vi "get waveplate status.vi"(8 "error in (no error)":errorcluster, 11 "Channel in":refnum<class "ECHARPE_Channel.lvclass">) -> (0 "error out":errorcluster, 2 "wp condition":string, 3 "Channel out":refnum<class "ECHARPE_Channel.lvclass">)   [LabVIEW 2018, in "ECHARPE_Channel.lvclass"]
uses:
  ECHARPE_Channel.lvclass
  Server/Server.lvclass/Server.ctl
  RxTx/RxTx.lvclass
  Server/Server.lvclass
panel:
  in  "Cluster":T1
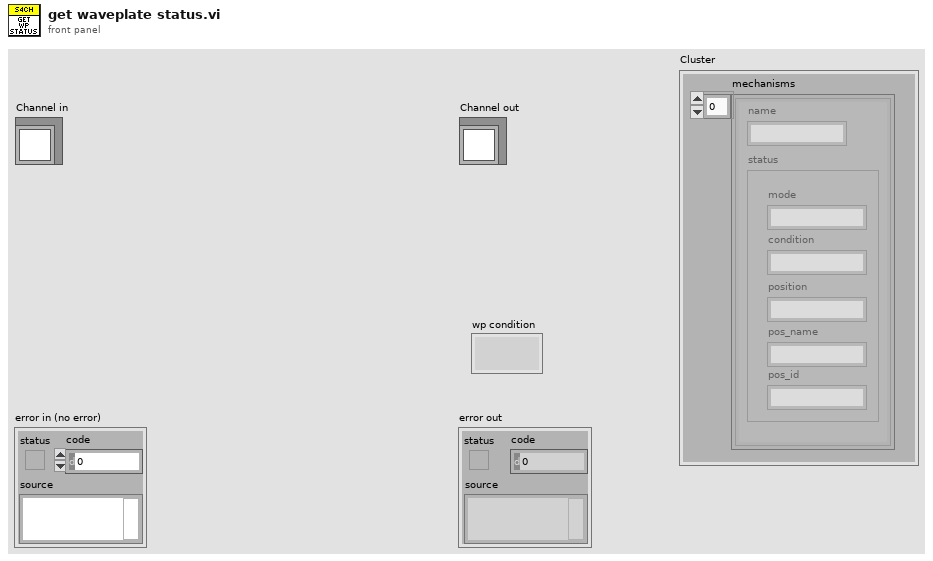
[diagram p1: front panel]
types:
  T1 = cluster{"mechanisms":cluster{"name":string, "status":cluster{"mode":string, "condition":string, "pos_name":string, "position":string, "pos_id":string}}[]}
  T2 = cluster{"State Machine.lvclass":refnum<class "State Machine.lvclass">, "RxTx.lvclass":refnum<class "RxTx.lvclass">, "Save_Header_RxTx.lvclass":refnum<class "RxTx.lvclass">, "Status SM.lvclass":refnum<class "State Machine.lvclass">, "Status RxTx.lvclass":refnum<class "RxTx.lvclass">, "servers array":refnum<class "Server.lvclass">[], "Events log file.lvclass":refnum<class "Log File.lvclass">, "Errors log file.lvclass":refnum<class "Log File.lvclass">, "Keywords log file.lvclass":refnum<class "Log File.lvclass">, "Sim_CCD.lvclass":refnum<class "Sim_CCD.lvclass">}
  T3 = cluster{"name":string, "status":cluster{"mode":string, "condition":string, "pos_name":string, "position":string, "pos_id":string}}[]
  T4 = cluster{"name":string, "status":cluster{"mode":string, "condition":string, "pos_name":string, "position":string, "pos_id":string}}
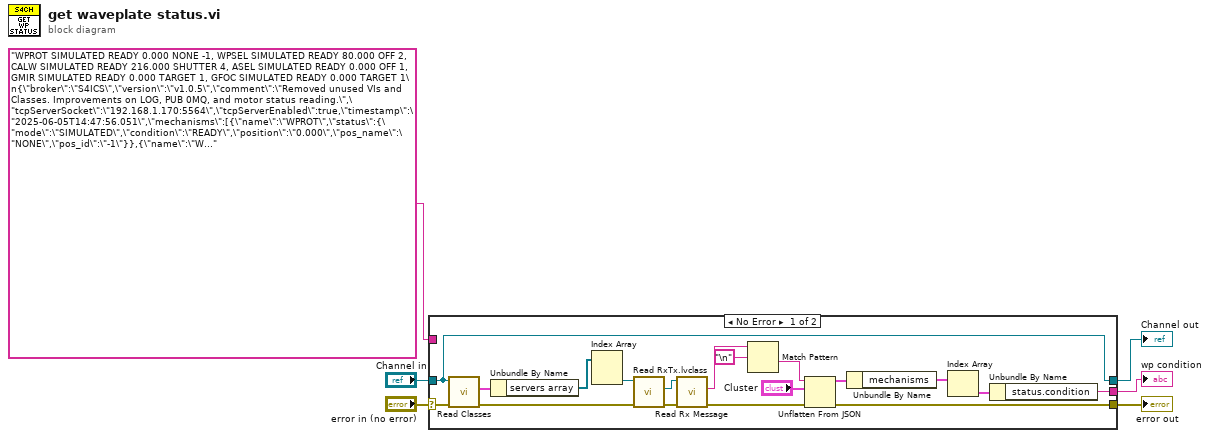
[diagram p0: block diagram]
diagram:
  n1 = case shown="No Error" "error in (no error)" {
    selector: "error in (no error)" -> [w11 w26]
    tunnel: [w24 w26] -> w5
    tunnel: [w10 w25] -> w3
    tunnel: "Channel in" -> [w10 w25]
    tunnel: [w14 _] -> w2
    tunnel: "WPROT SIMULATED READY 0.000 NONE -1, WPSEL SIMULATED READY 80.000 OFF 2, CALW SIMULATED READY 216.000 SHUTTER 4, ASEL SIMULATED READY 0.000 OFF 1, GMIR SIMULATED READY 0.000 TARGET 1, GFOC SIMULATED READY 0.000 TARGET 1\n{\"broker\":\"S4ICS\",\"version\":\"v1.0.5\",\"comment\":\"Removed unused VIs and Classes. Improvements on LOG, PUB 0MQ, and motor status reading.\",\"tcpServerSocket\":\"192.168.1.170:5564\",\"tcpServerEnabled\":true,\"timestamp\":\"2025-06-05T14:47:56.051\",\"mechanisms\":[{\"name\":\"WPROT\",\"status\":{\"mode\":\"SIMULATED\",\"condition\":\"READY\",\"position\":\"0.000\",\"pos_name\":\"NONE\",\"pos_id\":\"-1\"}},{\"name\":\"WPSEL\",\"status\":{\"mode\":\"SIMULATED\",\"condition\":\"READY\",\"position\":\"80.000\",\"pos_name\":\"OFF\",\"pos_id\":\"2\"}},{\"name\":\"CALW\",\"status\":{\"mode\":\"SIMULATED\",\"condition\":\"READY\",\"position\":\"216.000\",\"pos_name\":\"CLOSED\",\"pos_id\":\"4\"}},{\"name\":\"ASEL\",\"status\":{\"mode\":\"SIMULATED\",\"condition\":\"READY\",\"position\":\"0.000\",\"pos_name\":\"OFF\",\"pos_id\":\"1\"}},{\"name\":\"GMIR\",\"status\":{\"mode\":\"SIMULATED\",\"condition\":\"READY\",\"position\":\"0.000\",\"pos_name\":\"TARGET\",\"pos_id\":\"1\"}},{\"name\":\"GFOC\",\"status\":{\"mode\":\"SIMULATED\",\"condition\":\"READY\",\"position\":\"8.0\",\"pos_name\":\"TARGET\",\"pos_id\":\"-1\"}}]}" ("endpoint") -> [_ _]
    frame No Error {
      n2 = call-dynamic "Read Classes.vi"("error in (no error)"=w11, "Channel in"=w10) -> ("error out"=w7:errorcluster, "Classes"=w9:T2)  [unwired: 7 in, 1 out]
      n3 = Unbundle By Name(w9) -> ("servers array"=w8:refnum<class "Server.lvclass">[])
      n4 = Index Array(array=w8) -> (element #2=w21:refnum<class "Server.lvclass">)  [unwired: 2 in, 1 out]
      n5 = call "Read RxTx.lvclass.vi"("error in (no error)"=w7, "Server in"=w21) -> ("error out"=w22:errorcluster, "RxTx.lvclass"=w23:refnum<class "RxTx.lvclass">)  [unwired: 7 in, 1 out]
      n6 = call "Read Rx Message.vi"("error in (no error)"=w22, "RxTx in"=w23) -> ("error out"=w20:errorcluster, "Rx Message"=w12:string)  [unwired: 7 in, 1 out]
      n7 = Match Pattern(string=w12, regular expression="\n") -> (after substring=w13:string)  [unwired: 1 in, 3 out]
      n8 = Unflatten From JSON(JSON string=w13, type and defaults="Cluster", error in (no error)=w20) -> (value=w17:T1, error out=w24:errorcluster)  [unwired: 4 in]
      n9 = Unbundle By Name(w17) -> ("mechanisms"=w16:T3)
      n10 = Index Array(array=w16) -> (element=w15:T4)  [unwired: 1 in]
      n11 = Unbundle By Name(w15) -> ("status.condition"=w14:string)
    }
    frame Error {
    }
  }
  "error out" <- w5
  "Channel out" <- w3
  "wp condition" <- w2
